vi "Deadzone.vi"(1 "DeadZone":dbl, 2 "In":dbl) -> (0 "Out":dbl)   [LabVIEW 2019]
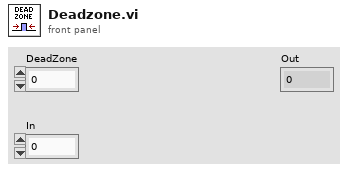
[diagram p1: front panel]
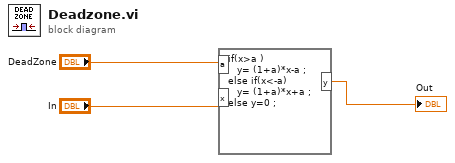
[diagram p0: block diagram]
diagram:
  n1 = formula code="if(x>a )\n   y= (1+a)*x-a ;\nelse if(x<-a)\n   y= (1+a)*x+a ;\nelse y=0 ;"("a"="DeadZone", "x"="In") -> ("y"=→"Out":dbl)
